vi "gmmregRegisterRedAndGreen.vi"() -> ()   [LabVIEW 2017]
panel:
  out "Image":T1(plugin-control)
  in  "manual":bool
  in  "ok":bool
  in  "temp_red":i32[](array[numeric])
  in  "adjust cut":i32=15
  out "size(s)":i32[](array[numeric])
  in  "#frames":i32=26
  in  "frame0":i32
  # "0. Set #frames to the number of galvo steps (N^2 + M)\n1. Select the single volume .dat file in the redgreen folder.\n2. Check that red and yellow dots overlap, more or less.\n3. Move in plane/frame index and check that the position of the\n    red spot is found correctly. When it's saturated, it's generally\n    a bit off from the actual center of the spot.\n3. Close."
  # "15"
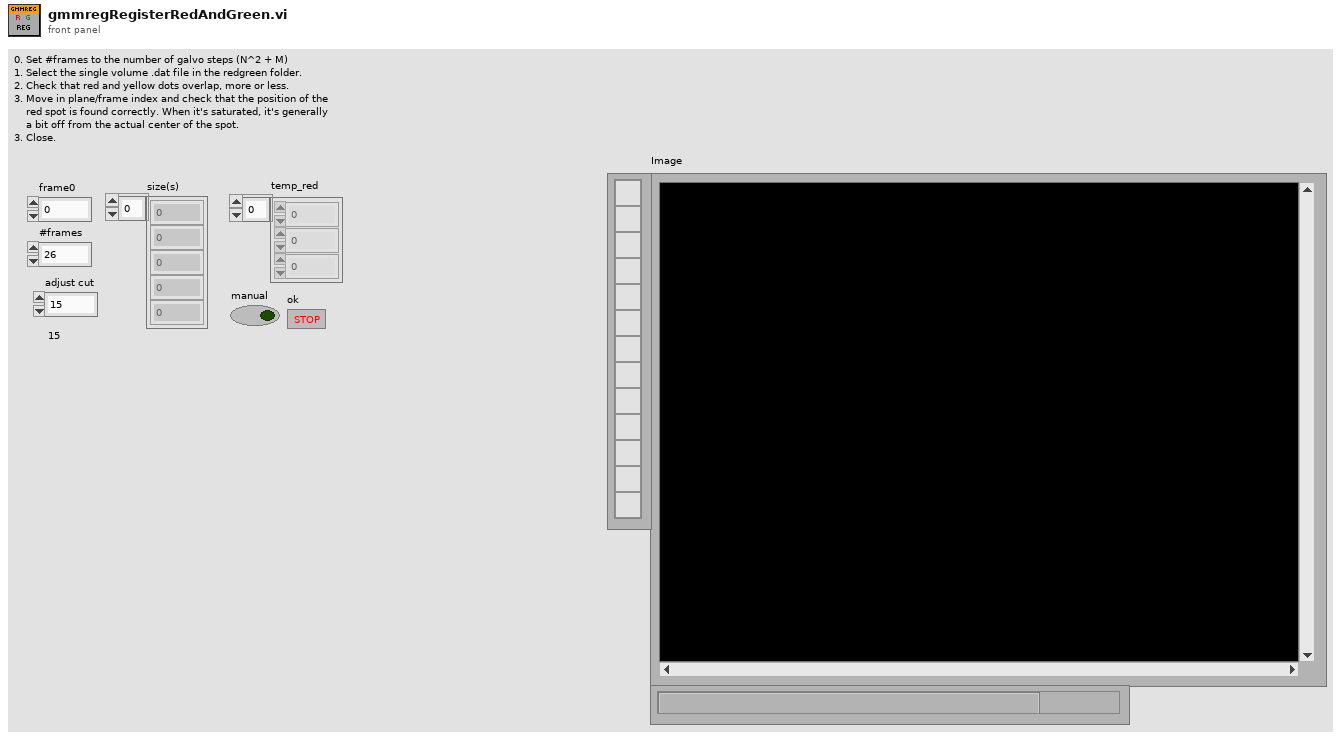
[diagram p1: front panel]
types:
  T1 = typedef "IMAQ Image.ctl" = refnum<image>
  T2 = typedef "Image Type" = u32
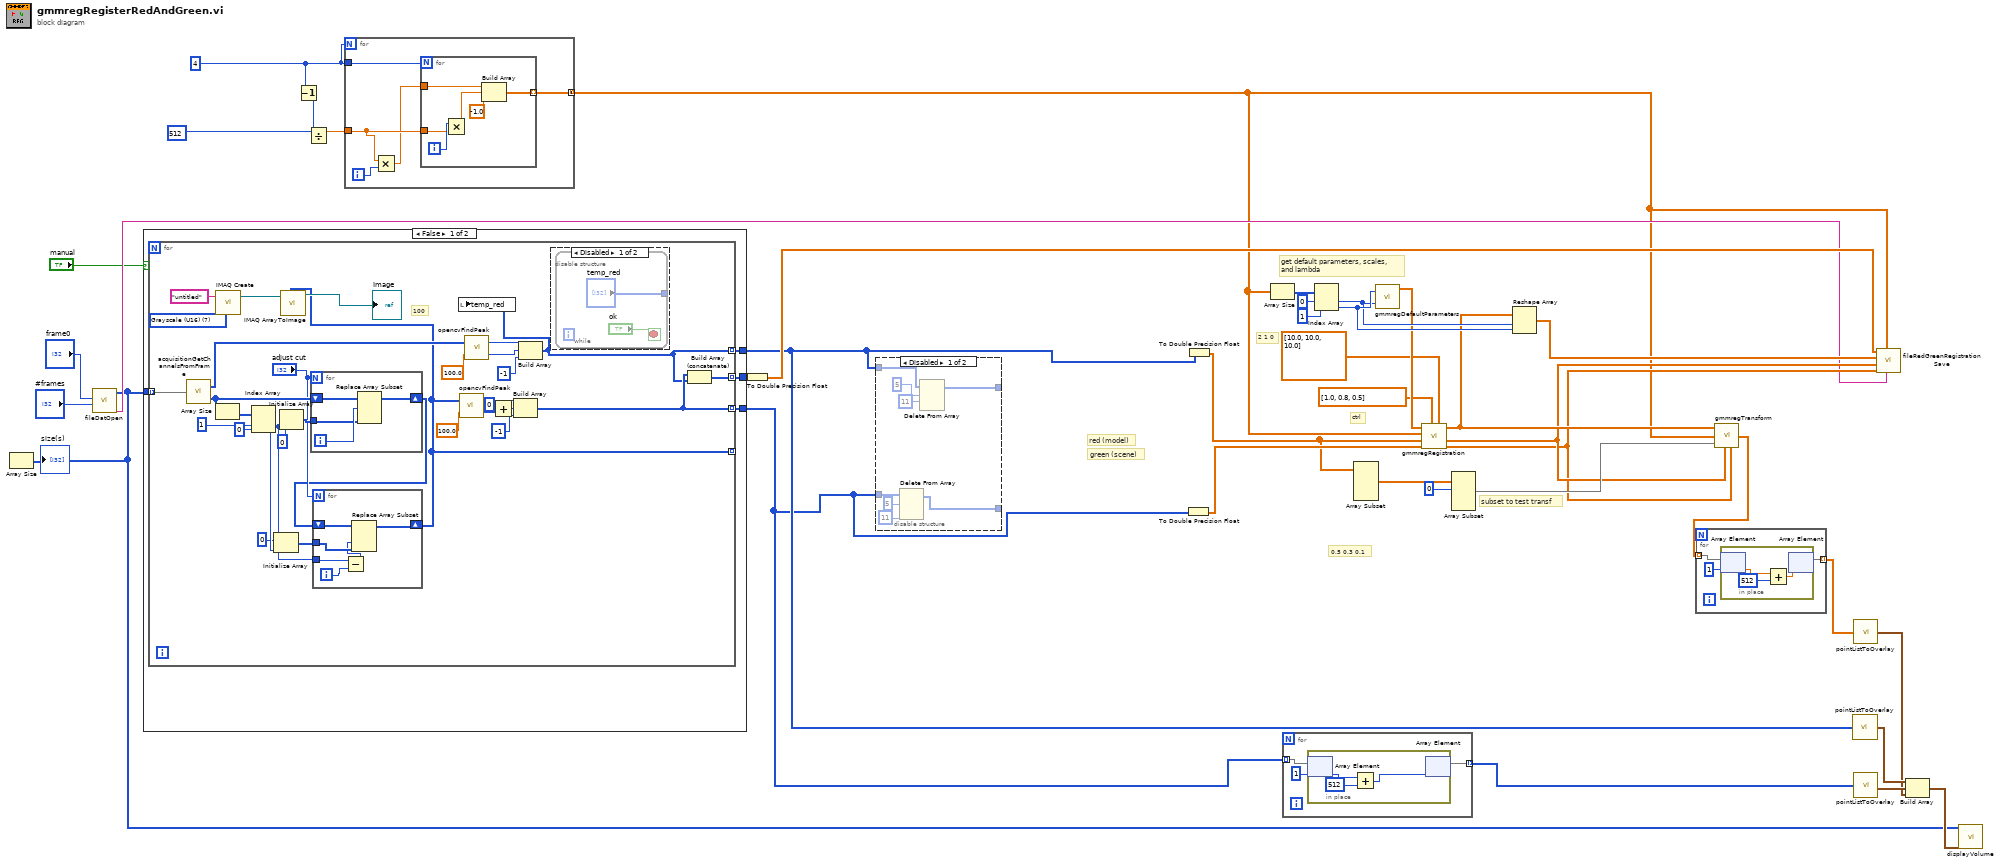
[diagram p0: block diagram]
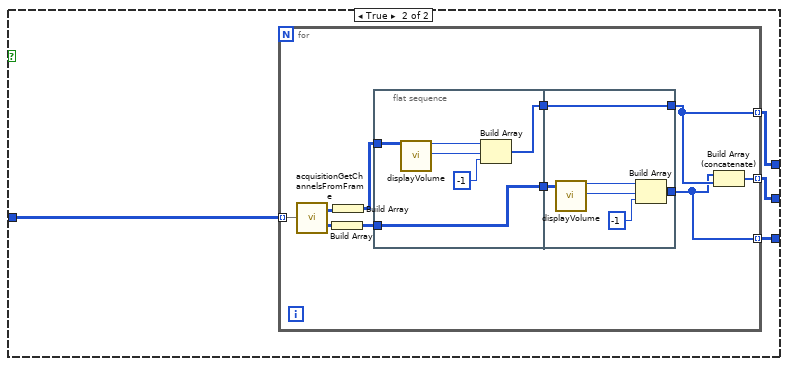
[diagram p4: hidden frame]
diagram:
  w9 = 4
  # "green (scene)"
  # "2 1 0"
  # "0.5 0.3 0.1"
  # "subset to test transf"
  # "ctrl"
  # "get default parameters, scales,\nand lambda"
  # "red (model)"
  n1 = call "fileDatOpen.vi"("#frames"="#frames", "frame0"="frame0") -> ("folder"=w13:string, "output array"=w4:u16[][][])  [unwired: 2 in, 2 out]
  n2 = Array Size(array=w4) -> (size(s)=→"size(s)":i32[])
  n3 = case shown="False" "manual" {
    tunnel: [w43 w89] -> w2
    tunnel: [w42 w90] -> w22
    tunnel: [w41 w88] -> w1
    tunnel: w4 -> [w40 w91]
    frame False {
      n4 = for {
        tunnel: w40 -> [w75] mode=indexing
        tunnel: [w66] -> w41 mode=indexing
        tunnel: [w45] -> _ mode=indexing
        tunnel: [w62] -> w43 mode=indexing
        tunnel: [w67] -> w42 mode=indexing
        w52 = T2 7 items=["Grayscale (U8)", "Grayscale (I16)", "Grayscale (SGL)", "Complex (CSG)", "RGB (U32)", "HSL (U32)", "RGB (U64)", "Grayscale (U16)"] ("Image Type")
        # "100"
        n5 = call "acquisitionGetChannelsFromFrame.vi"("frameIn"=w75) -> ("Red"=w68:u16[][], "Green"=w60:u16[][])
        n6 = Array Size(array=w60) -> (size(s)=w59:i32[])
        n7 = call "IMAQ Create"("Image Name"="untitled", "Image Type"=w52) -> ("New Image"=w54:T1)  [unwired: 3 in, 1 out]
        n8 = Index Array(array=w59, index #1=1 ("index"), index #2=0 ("index")) -> (element #1=w44:i32, element #2=w49:i32)
        n9 = Initialize Array(u16 0 ("element"), w49) -> (w47:u16[])
        n10 = Initialize Array(u16 0 ("element"), w44) -> (w56:u16[])
        n11 = for {
          N: "adjust cut" -> [_]
          tunnel: w56 -> [w83]
          shift-right: [w82] -> w46
          shift-left: w60 -> [w85]
          i -> [w84]
          n12 = Replace Array Subset(array=w85, new element=w83, index (row)=w84) -> (w82:u16[][])  [unwired: 1 in]
        }
        n13 = for {
          N: "adjust cut" -> [_]
          shift-right: [w79] -> w45
          shift-left: w46 -> [w81]
          tunnel: w47 -> [w80]
          tunnel: w44 -> [w78]
          i -> [w77]
          n14 = Subtract(x=w78, y=w77) -> (x-y=w76:i32)
          n15 = Replace Array Subset(array=w81, new element=w80, index (col)=w76) -> (w79:u16[][])  [unwired: 1 in]
        }
        n16 = call "IMAQ ArrayToImage"("Image Pixels (U16)"=w45, "Image"=w54) -> ("Image Out"=→"Image":T1)  [unwired: 8 in, 1 out]
        n17 = call "opencvFindPeak.vi"("blur"=100.0, "Image (2D)"=w45) -> ("maxLocY"=w64:i32, "maxLocX"=w65:i32)
        n18 = call "opencvFindPeak.vi"("blur"=100.0, "Image (2D)"=w68) -> ("maxLocY"=w70:i32, "maxLocX"=w69:i32)
        n19 = Add(x=0, y=w64) -> (x+y=w63:i32)
        n20 = Build Array(w65, w63, -1 ("element")) -> (w66:i32[])
        n21 = Build Array(w69, w70, -1 ("element")) -> (w62:i32[])
        n22 = local write "temp_red"(w62) -> ()
        n23 = disable-structure shown="Disabled" {
          frame Disabled {
            n24 = while {
              tunnel: ["temp_red"] -> _
              stop <- "ok" stop-if-true
            }
          }
          frame Enabled {
          }
        }
        n25 = Build Array (concatenate)(w66, w62) -> (w67:i32[])
      }
    }
    frame True {
      n26 = for {
        tunnel: w91 -> [w101] mode=indexing
        tunnel: [w94] -> w90 mode=indexing
        tunnel: [w93] -> w89 mode=indexing
        tunnel: [w92] -> w88 mode=indexing
        n27 = call "acquisitionGetChannelsFromFrame.vi"("frameIn"=w101) -> ("Red"=w100:u16[][], "Green"=w99:u16[][])
        n28 = Build Array(w99) -> (w95:u16[][][])
        n29 = Build Array(w100) -> (w98:u16[][][])
        n30 = flat-sequence {
          tunnel: w98 -> [w107]
          tunnel: [w105] -> w97
          tunnel: [w104] -> w96
          tunnel: w95 -> [w104]
          tunnel: [w113] -> w93
          tunnel: w97 -> [w113]
          tunnel: w96 -> [w111]
          tunnel: [w110] -> w92
          frame #0 {
            n31 = call "displayVolume.vi"("frames"=w107) -> ("X0out"=w103:i32, "Y0out"=w102:i32)  [unwired: 13 in, 4 out]
            n32 = Build Array(w103, w102, -1 ("element")) -> (w105:i32[])
          }
          frame #1 {
            n33 = call "displayVolume.vi"("frames"=w111) -> ("X0out"=w109:i32, "Y0out"=w108:i32)  [unwired: 13 in, 4 out]
            n34 = Build Array(w109, w108, -1 ("element")) -> (w110:i32[])
          }
        }
        n35 = Build Array (concatenate)(w92, w93) -> (w94:i32[])
      }
    }
  }
  n36 = Decrement(x=w9) -> (x-1=w8:i32)
  n37 = Divide(x=512, y=w8) -> (x/y=w11:dbl)
  n38 = for {
    N: w9 -> [_]
    tunnel: w9 -> [w118]
    tunnel: w11 -> [w116]
    tunnel: [w114] -> w12 mode=concatenating
    i -> [w117]
    n39 = Multiply(x=w116, y=w117) -> (x*y=w115:dbl)
    n40 = for {
      N: w118 -> [_]
      tunnel: w116 -> [w122]
      tunnel: w115 -> [w121]
      tunnel: [w119] -> w114 mode=indexing
      i -> [w123]
      n41 = Multiply(x=w123, y=w122) -> (x*y=w120:dbl)
      n42 = Build Array(w121, w120, -1.0 ("element")) -> (w119:dbl[])
    }
  }
  n43 = To Double Precision Float(number=w22) -> (double precision float=w21:dbl[][])
  n44 = disable-structure shown="Disabled" {
    disable-tunnel: w2 -> [w128 _]
    disable-tunnel: [w127 _] -> _
    disable-tunnel: w1 -> [w126 _]
    disable-tunnel: [w125 _] -> _
    frame Disabled {
      n45 = Delete From Array(array=w126, length=5, index (row)=11) -> (array with subset deleted=w125:i32[][])  [unwired: 1 in, 1 out]
      n46 = Delete From Array(array=w128, length=5, index (row)=11) -> (array with subset deleted=w127:i32[][])  [unwired: 1 in, 1 out]
    }
    frame Enabled {
    }
  }
  n47 = To Double Precision Float(number=w1) -> (double precision float=w29:dbl[][])
  n48 = To Double Precision Float(number=w2) -> (double precision float=w14:dbl[][])
  n49 = Array Size(array=w12) -> (size(s)=w34:i32[])
  n50 = for {
    tunnel: w1 -> [w135] mode=indexing
    tunnel: [w133] -> w17 mode=indexing
    n51 = in-place {
      n52 = in-place-array #1(w135, 1) -> (w138:i32)
      n53 = Add(x=w138, y=512) -> (x+y=w136:i32)
      n54 = in-place-array #1(w136) -> (w133:i32[])  [unwired: 1 out]
    }
  }
  n55 = Index Array(array=w34, index #1=0 ("index"), index #2=1 ("index")) -> (element #1=w36:i32, element #2=w37:i32)
  n56 = Array Subset(array=w14) -> (w27:dbl[][])  [unwired: 4 in]
  n57 = call "gmmregDefaultParameters.vi"("D (3)"=w37, "nctrlPts"=w36) -> ("param0"=w35:dbl[])  [unwired: 3 out]
  n58 = call "gmmregRegistration.vi"("lambda"=dbl[] [10.0, 10.0, 10.0], "scale"=dbl[] [1.0, 0.8, 0.5], "scene"=w29, "model"=w14, "ctrlPoints"=w12, "param0"=w35) -> ("denormParams out"=w18:dbl[], "normParams out"=w19:dbl[], "param0 out"=w28:dbl[])  [unwired: 2 in, 1 out]
  n59 = Array Subset(array=w27, index (row)=0 ("index")) -> (w25:dbl[][])  [unwired: 3 in]
  n60 = Reshape Array(w28, w36, w37) -> (w20:dbl[][])
  n61 = call "gmmregTransform.vi"("param0"=w28, "ctrlPts"=w12, "pts"=w25, "normParams"=w19, "denormParams"=w18) -> ("out"=w16:dbl[][])  [unwired: 4 in]
  n62 = for {
    tunnel: w16 -> [w141] mode=indexing
    tunnel: [w139] -> w15 mode=indexing
    n63 = in-place {
      n64 = in-place-array #2(w141, 1) -> (w144:dbl)
      n65 = Add(x=w144, y=512) -> (x+y=w142:dbl)
      n66 = in-place-array #2(w142) -> (w139:dbl[])  [unwired: 1 out]
    }
  }
  n67 = call "pointListToOverlay.vi"("points"=w2) -> ("overlay (XYZ)"=w38:cluster{"X":i32, "Y":i32, "Z":i32}[])
  n68 = call "pointListToOverlay.vi"("points"=w15) -> ("overlay (XYZ)"=w23:cluster{"X":i32, "Y":i32, "Z":i32}[])
  n69 = call "pointListToOverlay.vi"("points"=w17) -> ("overlay (XYZ)"=w39:cluster{"X":i32, "Y":i32, "Z":i32}[])
  n70 = call "fileRedGreenRegistrationSave.vi"("filesFolderName"=w13, "ctrl"=w12, "denormParam"=w18, "normParam"=w19, "param"=w20, "xy(green)xy(red)"=w21) -> ()  [unwired: 1 in]
  n71 = Build Array(w38, w39, w23) -> (w24:cluster{"X":i32, "Y":i32, "Z":i32}[][])
  n72 = call "displayVolume.vi"("frames"=w4, "overlay (z:-1 all planes)"=w24) -> ()  [unwired: 12 in, 6 out]
